vi "Pachube Check HTML Response LaunchPad.vi"(0 "HTML Response":string="HTTP/1.1 200 OK\r\nDate: Sat, 28 Mar 2009 22:52:16 GMT\r\nServer: hi\r\nLast-Modified: Sat, 28 Mar 2009 22:52:16 GMT\r\nStatus: 200 OK\r\nETag: \"f12402a1a587b0ebadc614d6f9dc9eb7\"\r\nPragma: no-cache\r\nCache-Control: no-cache, no-store, must-revalidate, pre-check=0, post-check=0\r\nContent-Type: application/xml; charset=utf-8\r\nContent-Length: 757\r\nExpires: Tue, 31 Mar 1981 05:00:00 GMT\r\nX-Revision: d29c0b9d3d976365bfb5a607be00fbfcd69a1fe4\r\nX-Transaction: 1238280736-91482-13826\r\nSet-Cookie: lang=; path=/\r\nSet-Cookie: _twitter_sess=BAh7CToJdXNlcmkE2%252FmgAToTcGFzc3dvcmRfdG9rZW4iLTkzZWM4NjI3YWZh%250AYzdmM2MwZmYzMjk2NGU2MDUyMDhmNzg1ZjM1ZTc6B2lkIiVlNGM5NGFjYjY2%250AN2QzYzM4ZjFjOWIzZWI2ZWFiYzE3MiIKZmxhc2hJQzonQWN0aW9uQ29udHJv%250AbGxlcjo6Rmxhc2g6OkZsYXNoSGFzaHsABjoKQHVzZWR7AA%253D%253D--5367941b0c0e984b065af3ce3acb181e1b013e10; domain=.twitter.com; path=/\r\nVary: Accept-Encoding\r\nConnection: close\r\n\r\n<?xml version=\"1.0\" encoding=\"UTF-8\"?>\n<status>\n  <created_at>Sat Mar 28 22:52:16 +0000 2009</created_at>\n  <id>1409287851</id>\n  <text>This is a test</text>\n  <source>web</source>\n  <truncated>false</truncated>\n  <in_reply_to_status_id></in_reply_to_status_id>\n  <in_reply_to_user_id></in_reply_to_user_id>\n  <favorited>false</favorited>\n  <in_reply_to_screen_name></in_reply_to_screen_name>\n  <user>\n    <id>27326939</id>\n    <name>Ian Bell</name>\n    <screen_name>zx99</screen_name>\n    <location></location>\n    <description></description>\n    <profile_image_url>http://static.twitter.com/images/default_profile_normal.png</profile_image_url>\n    <url></url>\n    <protected>false</protected>\n    <followers_count>0</followers_count>\n  </user>\n</status>\n", 1 "error in":errorcluster) -> (2 "Error":bool, 3 "Error code":i32, 4 "error out":errorcluster)   [LabVIEW 2010]
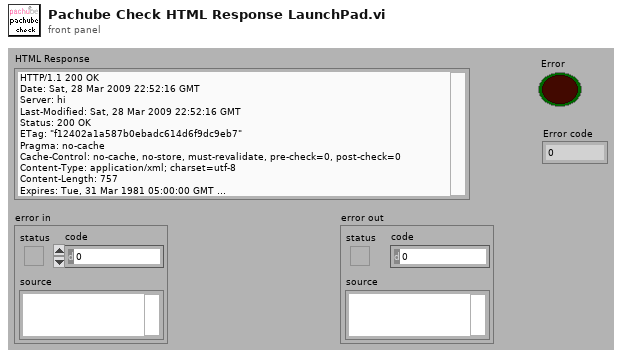
[diagram p1: front panel]
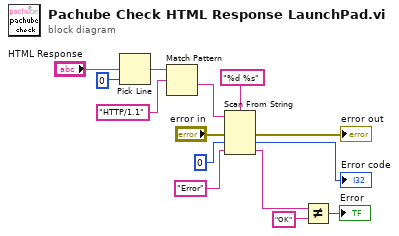
[diagram p0: block diagram]
diagram:
  n1 = Pick Line(multi-line string="HTML Response", line index=0) -> (output string=w11:string)  [unwired: 1 out]
  n2 = Match Pattern(string=w11, regular expression="HTTP/1.1") -> (after substring=w10:string)  [unwired: 4 out]
  n3 = Scan From String(format string="%d %s", input string=w10, error in="error in", default 1=0 ("default value 1"), default 2="Error" ("default value 2")) -> (error out=→"error out":errorcluster, output 1=→"Error code":i32, output 2=w6:string)  [unwired: 1 in, 2 out]
  n4 = Not Equal?(x=w6, y="OK") -> (x != y?=→"Error":bool)
